vi "Execute Route.vi"(8 "Robot location":dbl[](array[numeric]), 9 "Robot angle":dbl, 10 "Actual robot location":dbl[](array[numeric]), 11 "Route":dbl[][](array[numeric])) -> (0 "Succesful movemnet":bool, 1 "New grid robot location":dbl[](array[numeric]), 2 "New angle":dbl, 3 "New actaul robot location":dbl[](array[numeric]))   [LabVIEW 2015]
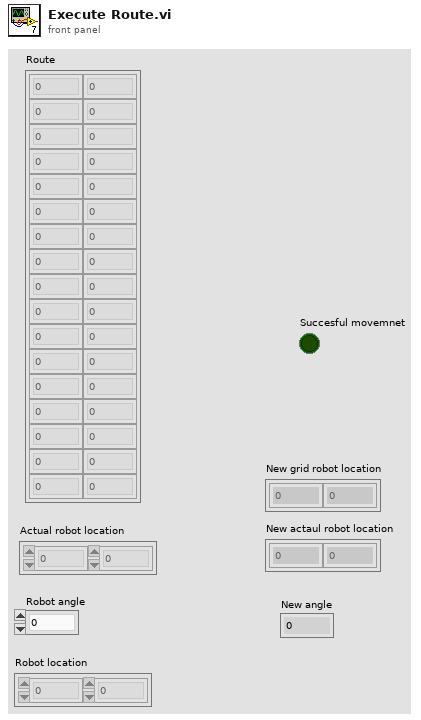
[diagram p1: front panel]
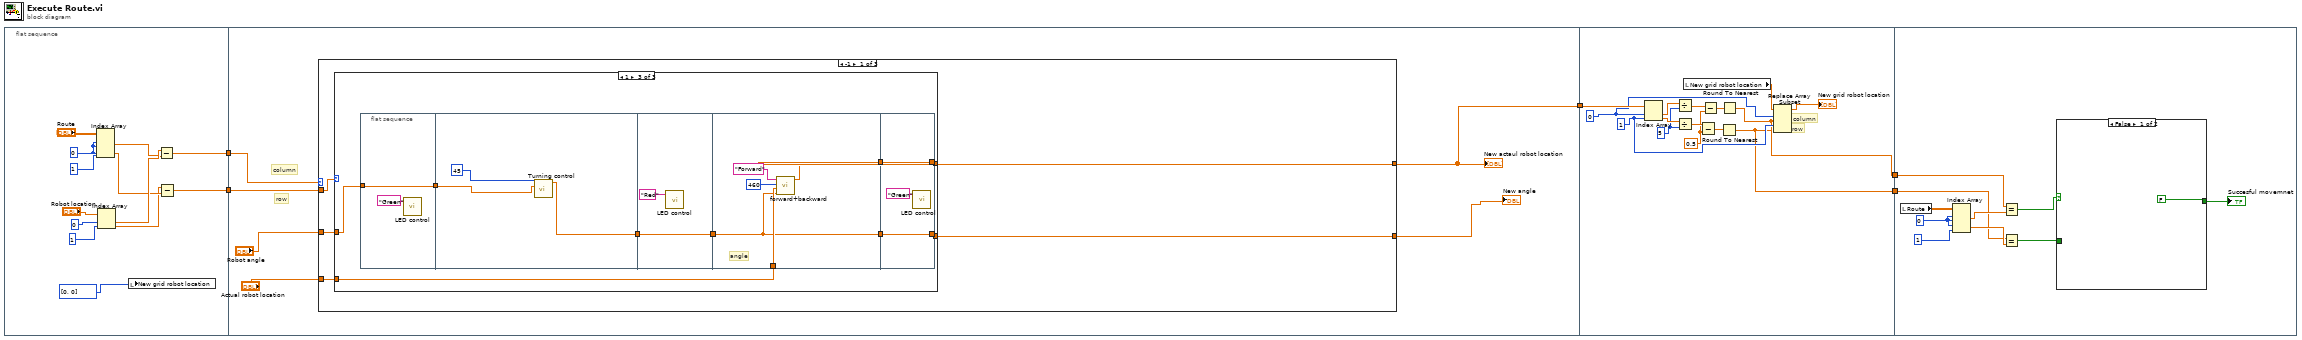
[diagram p0: block diagram]
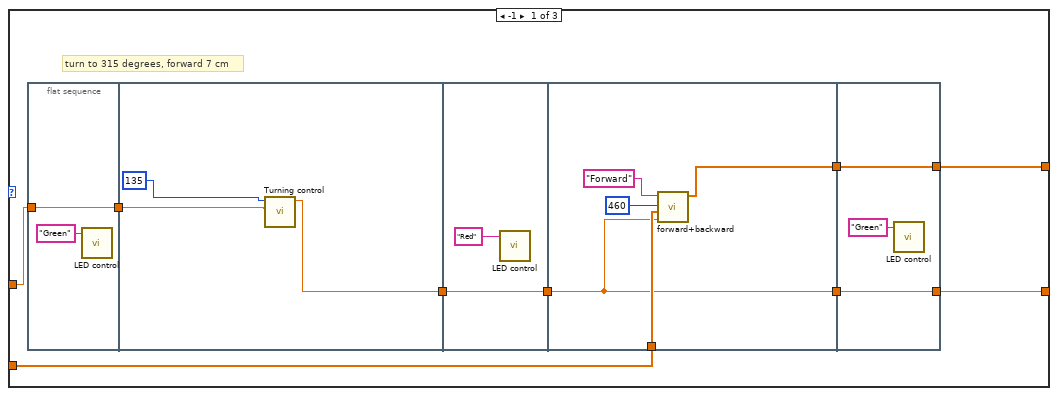
[diagram p2: hidden frame]
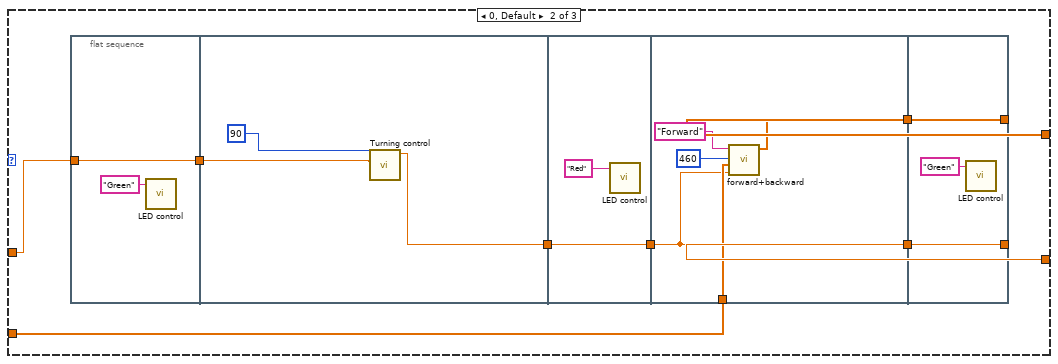
[diagram p3: hidden frame]
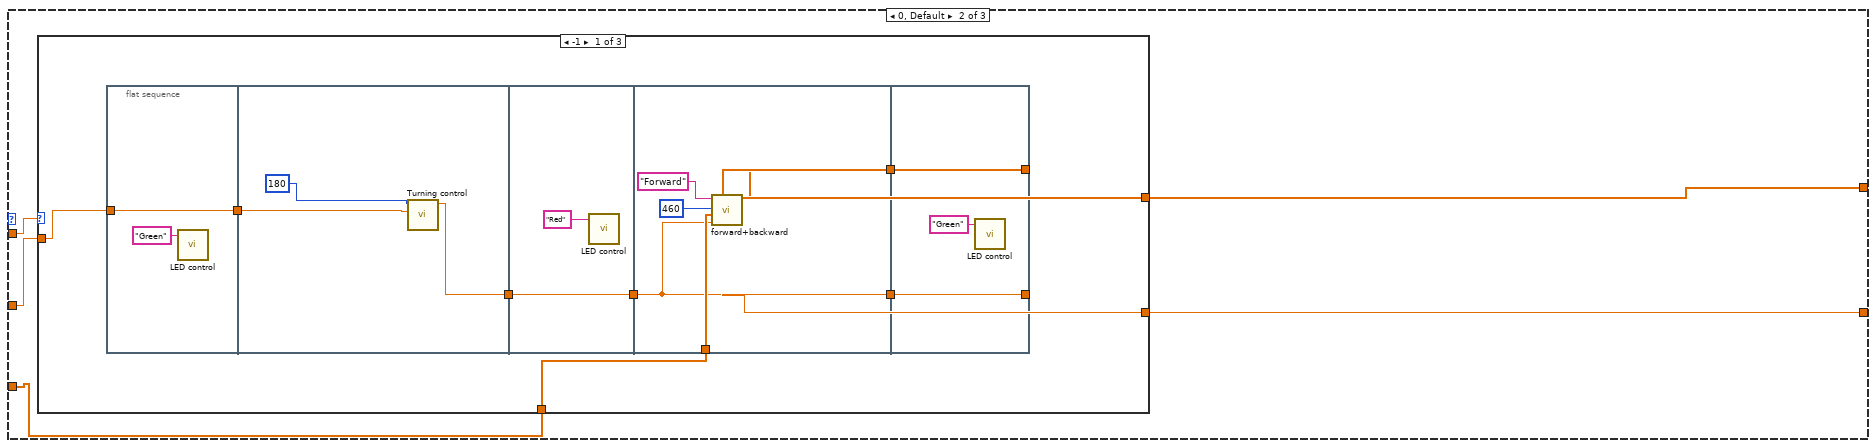
[diagram p4: hidden frame]
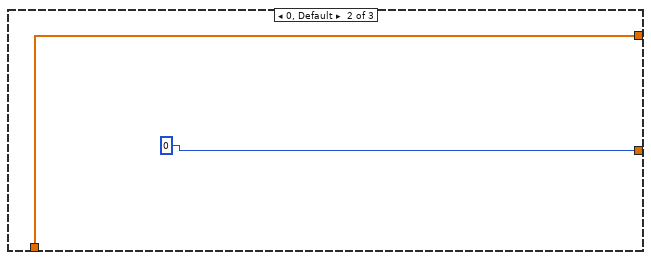
[diagram p5: hidden frame]
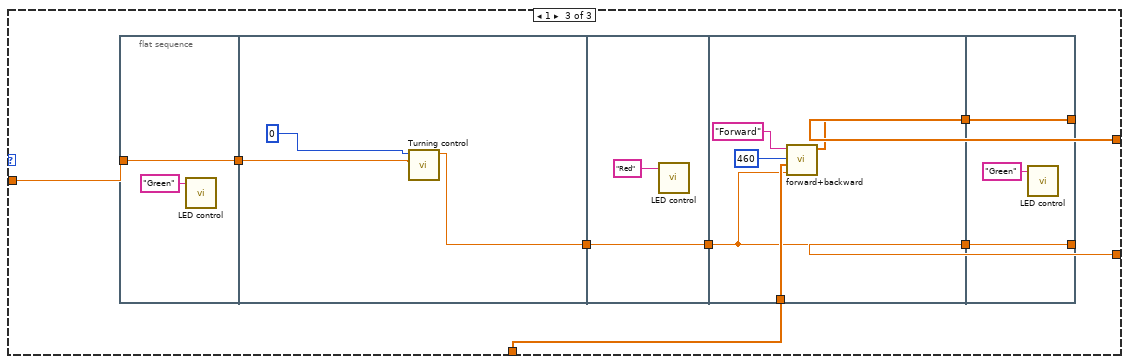
[diagram p6: hidden frame]
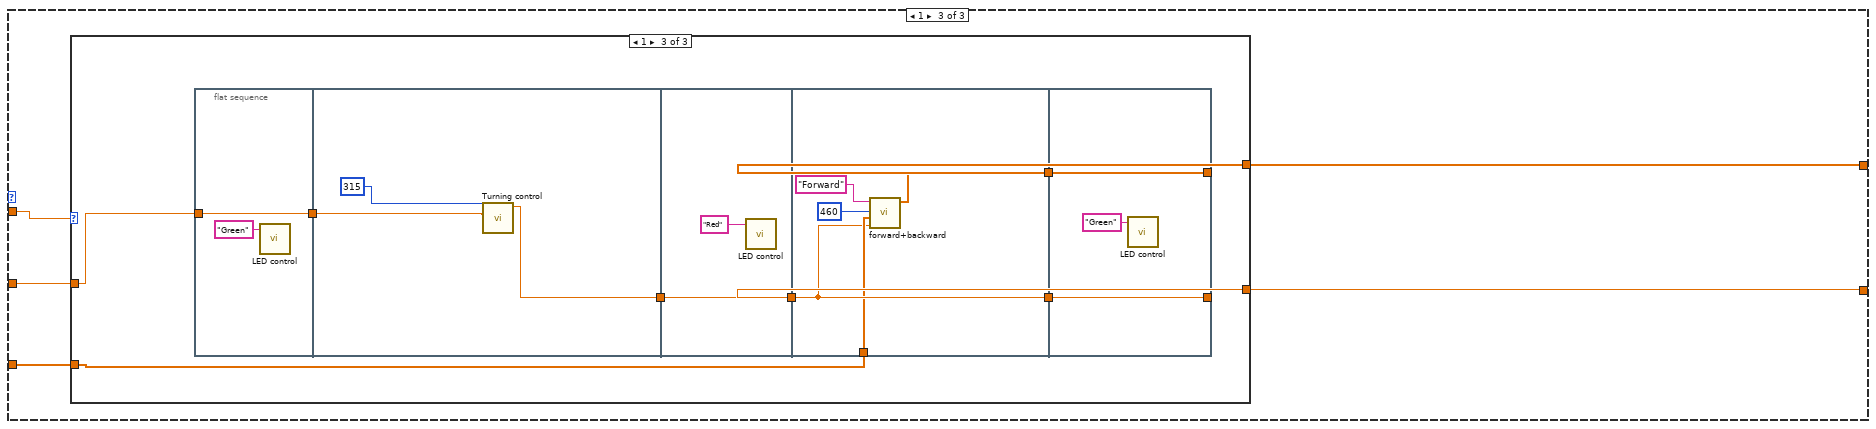
[diagram p7: hidden frame]
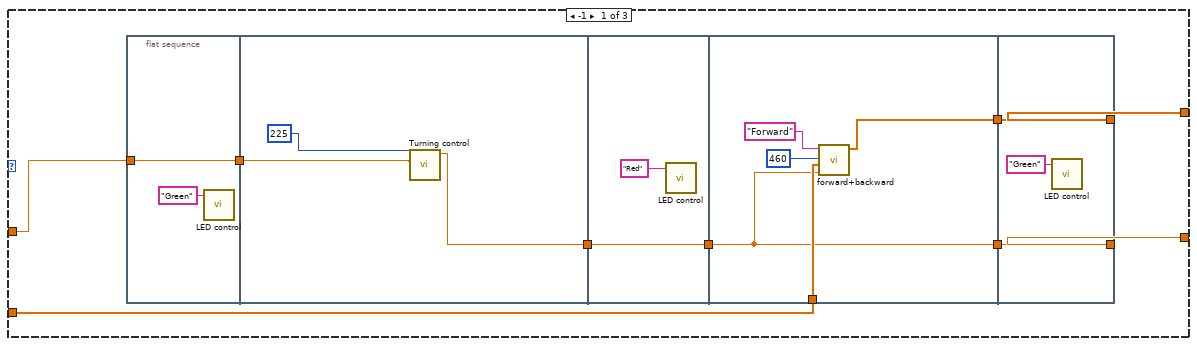
[diagram p8: hidden frame]
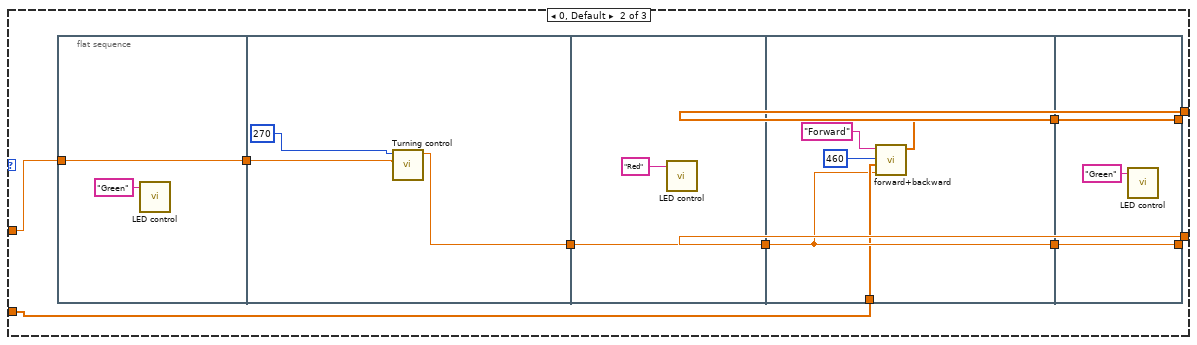
[diagram p9: hidden frame]
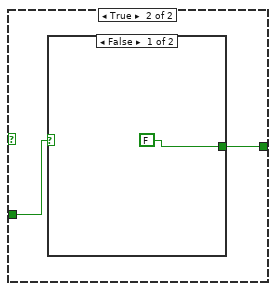
[diagram p10: hidden frame]
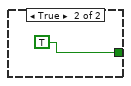
[diagram p11: hidden frame]
diagram:
  n1 = flat-sequence {
    tunnel: [w12] -> w5
    tunnel: [w11] -> w4
    tunnel: w5 -> [w24]
    tunnel: w4 -> [w23]
    tunnel: [w20] -> w3
    tunnel: w3 -> [w248]
    tunnel: [w235] -> w2
    tunnel: [w234] -> w1
    tunnel: w2 -> [w253]
    tunnel: w1 -> [w252]
    frame #0 {
      w16 = 0
      n2 = Index Array(array="Route", index (row) #1=w16, index (col) #1=w16, index (row) #2=w16, index (col) #2=1) -> (element #1=w9:dbl, element #2=w8:dbl)
      n3 = Index Array(array="Robot location", index #1=0, index #2=1) -> (element #1=w10:dbl, element #2=w7:dbl)
      n4 = local write "New grid robot location"(i32[] [0, 0]) -> ()
      n5 = Subtract(x=w10, y=w9) -> (x-y=w12:dbl)
      n6 = Subtract(x=w7, y=w8) -> (x-y=w11:dbl)
    }
    frame #1 {
      # "row"
      # "column"
      n7 = case shown="-1" w24 {
        tunnel: w23 -> [w29 w106 w161]
        tunnel: "Robot angle" -> [w28 w105 w160]
        tunnel: [w27 w103 w158] -> w19
        tunnel: [w26 w102 w157] -> w20
        tunnel: "Actual robot location" -> [w25 w104 w159]
        frame -1 {
          n8 = case shown="1" w29 {
            tunnel: w28 -> [w35 w54 w86]
            tunnel: [w38 w60 w84] -> w27
            tunnel: [w37 w61 w83] -> w26
            tunnel: w25 -> [w36 w62 w85]
            frame -1 {
              # "turn to 315 degrees, forward 7 cm"
              n9 = flat-sequence {
                tunnel: w35 -> [w40]
                tunnel: [w40] -> w34
                tunnel: [w43] -> w33
                tunnel: w34 -> [w42]
                tunnel: w33 -> [w45]
                tunnel: [w45] -> w32
                tunnel: w32 -> [w46]
                tunnel: w36 -> [w49]
                tunnel: [w46] -> w31
                tunnel: [w50] -> w30
                tunnel: [w52] -> w37
                tunnel: [w53] -> w38
                tunnel: w31 -> [w53]
                tunnel: w30 -> [w52]
                frame #0 {
                  n10 = call "LED control.vi"("RED/green"="Green") -> ()  [unwired: 11 in]
                }
                frame #1 {
                  n11 = call "Turning control.vi"("Robot angle"=w42, "Angle to move to"=135) -> ("Final Robot angle"=w43:dbl)  [unwired: 8 in]
                }
                frame #2 {
                  n12 = call "LED control.vi"("RED/green"="Red") -> ()  [unwired: 11 in]
                }
                frame #3 {
                  n13 = call "forward+backward.vi"("Robot angle"=w46, "Actual robot location"=w49, "wait time (ms)"=460, "Forward/backward"="Forward") -> ("New robot location"=w50:dbl[])  [unwired: 7 in]
                }
                frame #4 {
                  n14 = call "LED control.vi"("RED/green"="Green") -> ()  [unwired: 11 in]
                }
              }
            }
            frame 0, Default {
              n15 = flat-sequence {
                tunnel: w54 -> [w64]
                tunnel: [w64] -> w59
                tunnel: [w65] -> w58
                tunnel: w59 -> [w67]
                tunnel: w58 -> [w69]
                tunnel: [w69] -> w57
                tunnel: w57 -> [w70]
                tunnel: w62 -> [w73]
                tunnel: [w70] -> w56
                tunnel: [w74] -> w55
                tunnel: [w76] -> w61
                tunnel: [w77] -> w60
                tunnel: w56 -> [w77]
                tunnel: w55 -> [w76]
                frame #0 {
                  n16 = call "LED control.vi"("RED/green"="Green") -> ()  [unwired: 11 in]
                }
                frame #1 {
                  n17 = call "Turning control.vi"("Robot angle"=w67, "Angle to move to"=90) -> ("Final Robot angle"=w65:dbl)  [unwired: 8 in]
                }
                frame #2 {
                  n18 = call "LED control.vi"("RED/green"="Red") -> ()  [unwired: 11 in]
                }
                frame #3 {
                  n19 = call "forward+backward.vi"("Robot angle"=w70, "Actual robot location"=w73, "wait time (ms)"=460, "Forward/backward"="Forward") -> ("New robot location"=w74:dbl[])  [unwired: 7 in]
                }
                frame #4 {
                  n20 = call "LED control.vi"("RED/green"="Green") -> ()  [unwired: 11 in]
                }
              }
            }
            frame 1 {
              n21 = flat-sequence {
                tunnel: w86 -> [w88]
                tunnel: [w88] -> w82
                tunnel: [w91] -> w81
                tunnel: w82 -> [w90]
                tunnel: w81 -> [w93]
                tunnel: [w93] -> w80
                tunnel: w80 -> [w94]
                tunnel: w85 -> [w97]
                tunnel: [w94] -> w79
                tunnel: [w98] -> w78
                tunnel: [w100] -> w83
                tunnel: [w101] -> w84
                tunnel: w79 -> [w101]
                tunnel: w78 -> [w100]
                frame #0 {
                  n22 = call "LED control.vi"("RED/green"="Green") -> ()  [unwired: 11 in]
                }
                frame #1 {
                  n23 = call "Turning control.vi"("Robot angle"=w90, "Angle to move to"=45) -> ("Final Robot angle"=w91:dbl)  [unwired: 8 in]
                }
                frame #2 {
                  n24 = call "LED control.vi"("RED/green"="Red") -> ()  [unwired: 11 in]
                }
                frame #3 {
                  # "angle"
                  n25 = call "forward+backward.vi"("Robot angle"=w94, "Actual robot location"=w97, "wait time (ms)"=460, "Forward/backward"="Forward") -> ("New robot location"=w98:dbl[])  [unwired: 7 in]
                }
                frame #4 {
                  n26 = call "LED control.vi"("RED/green"="Green") -> ()  [unwired: 11 in]
                }
              }
            }
          }
        }
        frame 0, Default {
          n27 = case shown="-1" w106 {
            tunnel: w105 -> [w115 _ w141]
            tunnel: w104 -> [w114 w132 w140]
            tunnel: [w112 0 w138] -> w103
            tunnel: [w113 w132 w139] -> w102
            frame -1 {
              n28 = flat-sequence {
                tunnel: w115 -> [w117]
                tunnel: [w117] -> w111
                tunnel: [w120] -> w110
                tunnel: w111 -> [w119]
                tunnel: w110 -> [w122]
                tunnel: [w122] -> w109
                tunnel: w109 -> [w123]
                tunnel: w114 -> [w126]
                tunnel: [w123] -> w108
                tunnel: [w127] -> w107
                tunnel: [w129] -> w113
                tunnel: [w130] -> w112
                tunnel: w108 -> [w130]
                tunnel: w107 -> [w129]
                frame #0 {
                  n29 = call "LED control.vi"("RED/green"="Green") -> ()  [unwired: 11 in]
                }
                frame #1 {
                  n30 = call "Turning control.vi"("Robot angle"=w119, "Angle to move to"=180) -> ("Final Robot angle"=w120:dbl)  [unwired: 8 in]
                }
                frame #2 {
                  n31 = call "LED control.vi"("RED/green"="Red") -> ()  [unwired: 11 in]
                }
                frame #3 {
                  n32 = call "forward+backward.vi"("Robot angle"=w123, "Actual robot location"=w126, "wait time (ms)"=460, "Forward/backward"="Forward") -> ("New robot location"=w127:dbl[])  [unwired: 7 in]
                }
                frame #4 {
                  n33 = call "LED control.vi"("RED/green"="Green") -> ()  [unwired: 11 in]
                }
              }
            }
            frame 0, Default {
            }
            frame 1 {
              n34 = flat-sequence {
                tunnel: w141 -> [w143]
                tunnel: [w143] -> w137
                tunnel: [w146] -> w136
                tunnel: w137 -> [w145]
                tunnel: w136 -> [w148]
                tunnel: [w148] -> w135
                tunnel: w135 -> [w149]
                tunnel: w140 -> [w152]
                tunnel: [w149] -> w134
                tunnel: [w153] -> w133
                tunnel: [w155] -> w139
                tunnel: [w156] -> w138
                tunnel: w134 -> [w156]
                tunnel: w133 -> [w155]
                frame #0 {
                  n35 = call "LED control.vi"("RED/green"="Green") -> ()  [unwired: 11 in]
                }
                frame #1 {
                  n36 = call "Turning control.vi"("Robot angle"=w145, "Angle to move to"=0) -> ("Final Robot angle"=w146:dbl)  [unwired: 8 in]
                }
                frame #2 {
                  n37 = call "LED control.vi"("RED/green"="Red") -> ()  [unwired: 11 in]
                }
                frame #3 {
                  n38 = call "forward+backward.vi"("Robot angle"=w149, "Actual robot location"=w152, "wait time (ms)"=460, "Forward/backward"="Forward") -> ("New robot location"=w153:dbl[])  [unwired: 7 in]
                }
                frame #4 {
                  n39 = call "LED control.vi"("RED/green"="Green") -> ()  [unwired: 11 in]
                }
              }
            }
          }
        }
        frame 1 {
          n40 = case shown="1" w161 {
            tunnel: w160 -> [w170 w194 w210]
            tunnel: w159 -> [w169 w193 w218]
            tunnel: [w168 w192 w217] -> w158
            tunnel: [w167 w191 w216] -> w157
            frame -1 {
              n41 = flat-sequence {
                tunnel: w170 -> [w172]
                tunnel: [w172] -> w166
                tunnel: [w175] -> w165
                tunnel: w166 -> [w173]
                tunnel: w165 -> [w177]
                tunnel: [w177] -> w164
                tunnel: w164 -> [w178]
                tunnel: w169 -> [w181]
                tunnel: [w178] -> w163
                tunnel: [w182] -> w162
                tunnel: [w184] -> w167
                tunnel: [w185] -> w168
                tunnel: w163 -> [w185]
                tunnel: w162 -> [w184]
                frame #0 {
                  n42 = call "LED control.vi"("RED/green"="Green") -> ()  [unwired: 11 in]
                }
                frame #1 {
                  n43 = call "Turning control.vi"("Robot angle"=w173, "Angle to move to"=225) -> ("Final Robot angle"=w175:dbl)  [unwired: 8 in]
                }
                frame #2 {
                  n44 = call "LED control.vi"("RED/green"="Red") -> ()  [unwired: 11 in]
                }
                frame #3 {
                  n45 = call "forward+backward.vi"("Robot angle"=w178, "Actual robot location"=w181, "wait time (ms)"=460, "Forward/backward"="Forward") -> ("New robot location"=w182:dbl[])  [unwired: 7 in]
                }
                frame #4 {
                  n46 = call "LED control.vi"("RED/green"="Green") -> ()  [unwired: 11 in]
                }
              }
            }
            frame 0, Default {
              n47 = flat-sequence {
                tunnel: w194 -> [w196]
                tunnel: [w196] -> w190
                tunnel: [w199] -> w189
                tunnel: w190 -> [w197]
                tunnel: w189 -> [w201]
                tunnel: [w201] -> w188
                tunnel: w188 -> [w202]
                tunnel: w193 -> [w205]
                tunnel: [w202] -> w187
                tunnel: [w206] -> w186
                tunnel: [w208] -> w191
                tunnel: [w209] -> w192
                tunnel: w187 -> [w209]
                tunnel: w186 -> [w208]
                frame #0 {
                  n48 = call "LED control.vi"("RED/green"="Green") -> ()  [unwired: 11 in]
                }
                frame #1 {
                  n49 = call "Turning control.vi"("Robot angle"=w197, "Angle to move to"=270) -> ("Final Robot angle"=w199:dbl)  [unwired: 8 in]
                }
                frame #2 {
                  n50 = call "LED control.vi"("RED/green"="Red") -> ()  [unwired: 11 in]
                }
                frame #3 {
                  n51 = call "forward+backward.vi"("Robot angle"=w202, "Actual robot location"=w205, "wait time (ms)"=460, "Forward/backward"="Forward") -> ("New robot location"=w206:dbl[])  [unwired: 7 in]
                }
                frame #4 {
                  n52 = call "LED control.vi"("RED/green"="Green") -> ()  [unwired: 11 in]
                }
              }
            }
            frame 1 {
              n53 = flat-sequence {
                tunnel: w210 -> [w220]
                tunnel: [w220] -> w215
                tunnel: [w223] -> w214
                tunnel: w215 -> [w221]
                tunnel: w214 -> [w225]
                tunnel: [w225] -> w213
                tunnel: w213 -> [w226]
                tunnel: w218 -> [w229]
                tunnel: [w226] -> w212
                tunnel: [w230] -> w211
                tunnel: [w232] -> w216
                tunnel: [w233] -> w217
                tunnel: w212 -> [w233]
                tunnel: w211 -> [w232]
                frame #0 {
                  n54 = call "LED control.vi"("RED/green"="Green") -> ()  [unwired: 11 in]
                }
                frame #1 {
                  n55 = call "Turning control.vi"("Robot angle"=w221, "Angle to move to"=315) -> ("Final Robot angle"=w223:dbl)  [unwired: 8 in]
                }
                frame #2 {
                  n56 = call "LED control.vi"("RED/green"="Red") -> ()  [unwired: 11 in]
                }
                frame #3 {
                  n57 = call "forward+backward.vi"("Robot angle"=w226, "Actual robot location"=w229, "wait time (ms)"=460, "Forward/backward"="Forward") -> ("New robot location"=w230:dbl[])  [unwired: 7 in]
                }
                frame #4 {
                  n58 = call "LED control.vi"("RED/green"="Green") -> ()  [unwired: 11 in]
                }
              }
            }
          }
        }
      }
      "New actaul robot location" <- w20
      "New angle" <- w19
    }
    frame #2 {
      w242 = 0.5
      w245 = 5
      w236 = 1
      w237 = 0
      # "column"
      # "row"
      n59 = Index Array(array=w248, index #1=w237, index #2=w236) -> (element #1=w247:dbl, element #2=w246:dbl)
      n60 = Divide(x=w247, y=w245) -> (x/y=w244:dbl)
      n61 = Divide(x=w246, y=w245) -> (x/y=w243:dbl)
      n62 = local read "New grid robot location"() -> (w238:dbl[])
      n63 = Subtract(x=w243, y=w242) -> (x-y=w240:dbl)
      n64 = Subtract(x=w244, y=w242) -> (x-y=w241:dbl)
      n65 = Round To Nearest(number=w240) -> (nearest integer value=w234:dbl)
      n66 = Round To Nearest(number=w241) -> (nearest integer value=w235:dbl)
      n67 = Replace Array Subset(array=w238, new element #1=w235, index #1=w237, new element #2=w234, index #2=w236) -> (→"New grid robot location":dbl[])
    }
    frame #3 {
      w256 = 0
      n68 = local read "Route"() -> (w254:dbl[][])
      n69 = Index Array(array=w254, index (row) #1=w256, index (col) #1=w256, index (row) #2=w256, index (col) #2=1) -> (element #1=w258:dbl, element #2=w257:dbl)
      n70 = Equal?(x=w253, y=w258) -> (x = y?=w251:bool)
      n71 = Equal?(x=w252, y=w257) -> (x = y?=w250:bool)
      n72 = case shown="False" w251 {
        tunnel: w250 -> [_ w261]
        tunnel: [FALSE w260] -> w249
        frame False {
        }
        frame True {
          n73 = case shown="False" w261 {
            tunnel: [FALSE TRUE] -> w260
            frame False {
            }
            frame True {
            }
          }
        }
      }
      "Succesful movemnet" <- w249
    }
  }
